vi "Main VI.vi"() -> ()   [LabVIEW 2010]
panel:
  in  "stop":bool
  in  "OpenWinThree":bool
  in  "OpenWinTwo":bool
  in  "OpenWinOne":bool
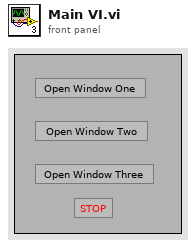
[diagram p1: front panel]
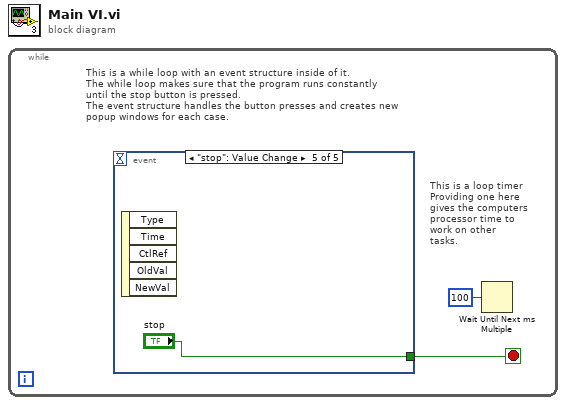
[diagram p0: block diagram]
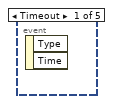
[diagram p2: hidden frame]
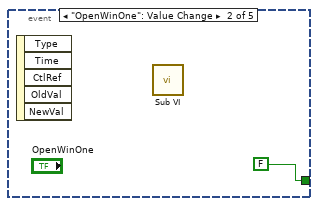
[diagram p3: hidden frame]
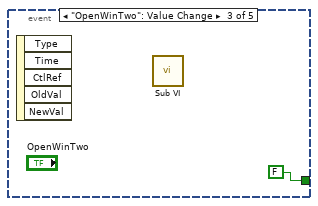
[diagram p4: hidden frame]
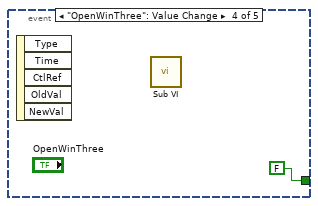
[diagram p5: hidden frame]
diagram:
  n1 = while {
    stop <- w1 stop-if-true
    # "This is a loop timer\nProviding one here\ngives the computers\nprocessor time to\nwork on other\ntasks."
    # "This is a while loop with an event structure inside of it. \nThe while loop makes sure that the program runs constantly \nuntil the stop button is pressed.\nThe event structure handles the button presses and creates new \npopup windows for each case."
    n2 = event shown="[4] \"stop\": Value Change" {
      selector: _ -> [_ _ _ _ _]
      dyn-events: _ -> [_ _ _ _ _]
      timeout: _ -> [_ _ _ _ _]
      tunnel: [_ FALSE FALSE FALSE "stop"] -> w1
      event Timeout {
        n3 = event-data() -> ()  [unwired: 1 in, 2 out]
      }
      event "OpenWinOne": Value Change {
        n4 = event-data() -> ()  [unwired: 1 in, 5 out]
        n5 = call "Sub VI.vi"() -> ()  [unwired: 12 in]
      }
      event "OpenWinTwo": Value Change {
        n6 = event-data() -> ()  [unwired: 1 in, 5 out]
        n7 = call "Sub VI.vi"() -> ()  [unwired: 12 in]
      }
      event "OpenWinThree": Value Change {
        n8 = event-data() -> ()  [unwired: 1 in, 5 out]
        n9 = call "Sub VI.vi"() -> ()  [unwired: 12 in]
      }
      event "stop": Value Change {
        n10 = event-data() -> ()  [unwired: 1 in, 5 out]
      }
    }
    n11 = Wait Until Next ms Multiple(millisecond multiple=u32 100) -> ()  [unwired: 1 out]
  }
